vi "Position_Show.vi"(3 "Image Out 4":T1, 4 "Group 2":string, 5 "数值":dbl, 6 "NewNodeM 2":cluster{"NewNodeM[0]":dbl, "NewNodeM[1]":dbl}) -> (1 "Image Out 3":T1)   [LabVIEW 2014]
doc: "根据轨迹坐标点数据画椭圆"
uses:
  <vilib>/vision/Image Controls.llb/IMAQ Image.ctl
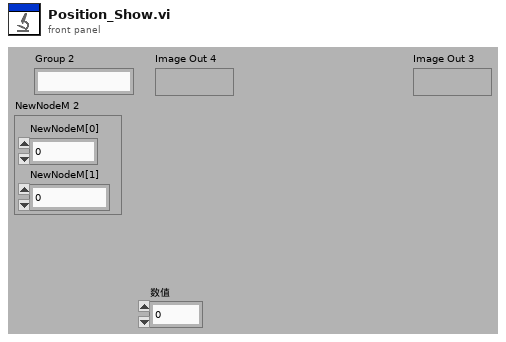
[diagram p1: front panel]
types:
  T1 = typedef "IMAQ Image.ctl" = refnum<image>
  T2 = cluster{"NewNodeM[0]":dbl, "NewNodeM[1]":dbl, "NewNodeM[0]":dbl, "NewNodeM[1]":dbl}
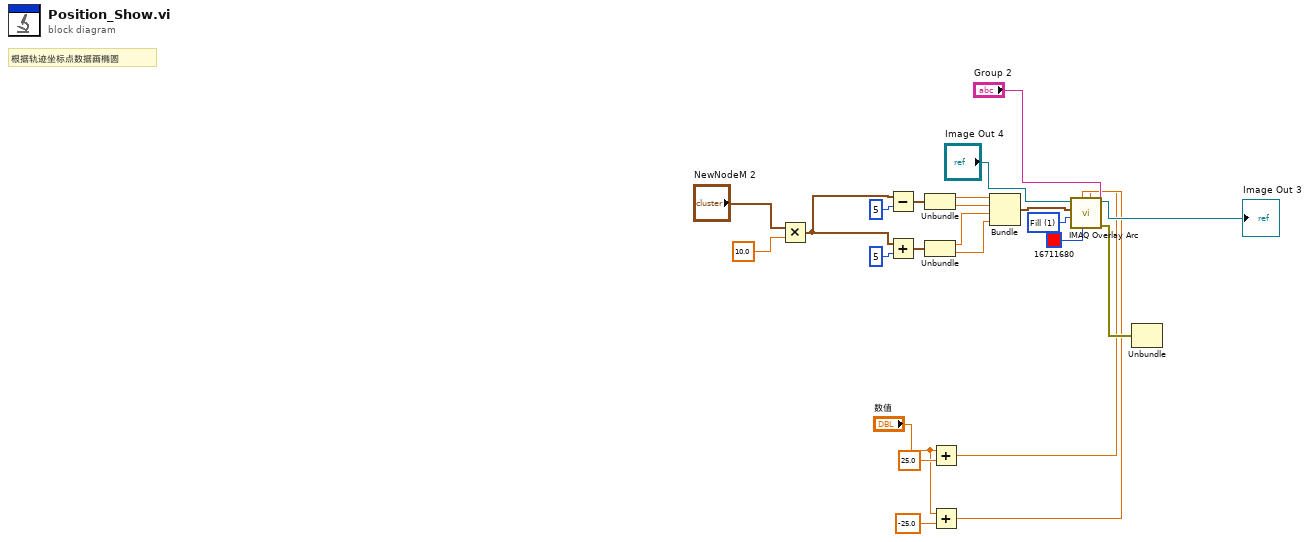
[diagram p0: block diagram]
diagram:
  w13 = u32 1 items=["Frame", "Fill"] ("Drawing Mode (Frame)")
  # "根据轨迹坐标点数据画椭圆"
  n1 = Multiply(x="NewNodeM 2", y=10.0 ("NewNodeM[0]")) -> (x*y=w23:cluster{"NewNodeM[0]":dbl, "NewNodeM[1]":dbl})
  n2 = Subtract(x=w23, y=u32 5 ("等待时间（毫秒）")) -> (x-y=w16:cluster{"NewNodeM[0]":dbl, "NewNodeM[1]":dbl})
  n3 = Add(x=w23, y=u32 5 ("等待时间（毫秒）")) -> (x+y=w17:cluster{"NewNodeM[0]":dbl, "NewNodeM[1]":dbl})
  n4 = Unbundle(w16) -> ("NewNodeM[0]"=w15:dbl, "NewNodeM[1]"=w3:dbl)
  n5 = Unbundle(w17) -> ("NewNodeM[0]"=w14:dbl, "NewNodeM[1]"=w2:dbl)
  n6 = Add(x="数值", y=25.0) -> (x+y=w4:dbl)
  n7 = Add(x="数值", y=-25.0) -> (x+y=w5:dbl)
  n8 = Bundle("NewNodeM[0]"=w15, "NewNodeM[1]"=w3, "NewNodeM[0]"=w14, "NewNodeM[1]"=w2) -> (w1:T2)  [unwired: 1 in]
  n9 = call "IMAQ Overlay Arc"("Group"="Group 2", "End Angle (degrees)"=w4, "Color"=u32 16711680, "Start Angle (degrees)"=w5, "Drawing Mode (Frame)"=w13, "Bounding Rectangle"=w1, "Image"="Image Out 4") -> ("error out"=w9:errorcluster, "Image Out"=→"Image Out 3":T1)  [unwired: 3 in]
  n10 = Unbundle(w9) -> ()  [unwired: 3 out]
